vi "Local2Global Target Values.vi"(6 "Direction":enum16{" +", " - "}(ring)=enum." - ", 11 "Target  Inputs":T1[](array[typedef])) -> (3 "Target  Outputs":T1[](array[typedef]))   [LabVIEW 2009]
uses:
  MixedMode/Messages/Target.ctl
  Data Access Objects/Metadata/LBCB Number.ctl
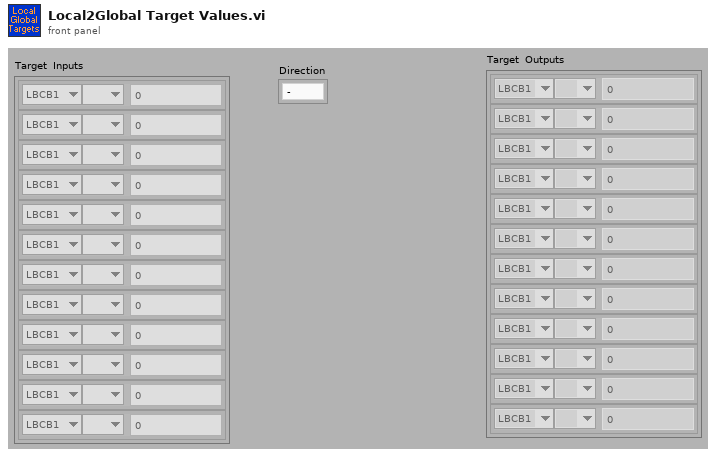
[diagram p1: front panel]
types:
  T1 = typedef "Target.ctl" = cluster{"LBCB Number":T2, "DOF Vectors":enum16{" ", "Dx", "Dy", "Dz", "Rx", "Ry", "Rz", "Fx", "Fy", "Fz", "Mx", "My", "Mz"}, "Amount":dbl}
  T2 = typedef "LBCB Number.ctl" = enum16{"LBCB1", "LBCB2"}
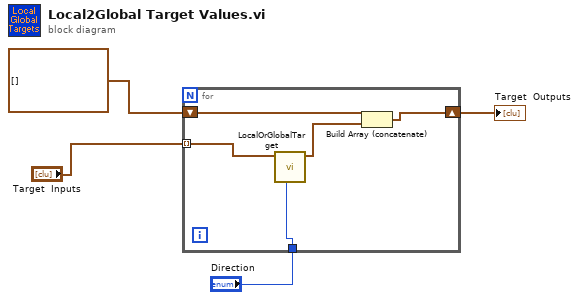
[diagram p0: block diagram]
diagram:
  n1 = for {
    tunnel: "Target  Inputs" -> [w9] mode=indexing
    shift-right: [w6] -> w2
    shift-left: T1[] [] -> [w7]
    tunnel: "Direction" -> [w5]
    n2 = call "LocalOrGlobalTarget.vi"("Direction"=w5, "Target"=w9) -> ("Adjusted Target"=w8:T1)  [unwired: 9 in]
    n3 = Build Array (concatenate)(w7, w8) -> (w6:T1[])
  }
  "Target  Outputs" <- w2
